vi "Robot Global Data.vi"() -> ()   [LabVIEW 2016]
doc: "This global VI can contain as many global variables as you need. Place a control on the panel, give it a good name. To read or write to it from a VI, drag the icon to the diagram of that VI. You can also drag from the project. Click on the node to change which global you access. You shouldn't have multiple locations writing to a global or it will cause a race-condition."
uses:
  <vilib>/Rock Robotics/WPI/Camera/WPI_CameraImageSize.ctl
  <vilib>/Rock Robotics/WPI/DriverStation/WPI_DriverStationRobotMode2.ctl
  Common Code/Dashboard Control Data.ctl
  Common Code/Drivetrain Settings.ctl
  Common Code/PID Gains.ctl
  Common Code/Input Modifier.ctl
  Common Code/Intake Presets.ctl
  Common Code/Shooter Presets.ctl
  Common Code/Vision Target Packet.ctl
  Common Code/Drivetrain Encoder Values.ctl
  Common Code/Encoder Values.ctl
  Common Code/Auto Agitator Settings.ctl
  Common Code/Climber Settings.ctl
  Common Code/LED Global Data.ctl
  Common Code/Drivetrain Command Cluster.ctl
  Common Code/Drivetrain Mode.ctl
  Common Code/Intake Control Cluster.ctl
  Common Code/Intake Modes.ctl
  Common Code/Intake Auto States.ctl
  Common Code/Intake Trip States.ctl
  Common Code/Keyboard Packet.ctl
  Common Code/Manual Command Cluster.ctl
  Common Code/Shooter Control Cluster'.ctl
  Common Code/Shooter Modes.ctl
  Common Code/Shooter Commands.ctl
  Common Code/Manual Shoot Cluster.ctl
  Common Code/Shot Type.ctl
  Common Code/Auton File Lists.ctl
  Common Code/Auton Command Cluster.ctl
  Common Code/Climb Command Cluster.ctl
  Common Code/Drivetrain Status Cluster.ctl
  Common Code/Intake Status Cluster.ctl
  Common Code/Climb Status Cluster.ctl
  Common Code/Shooter Status Cluster.ctl
  Common Code/Dashboard Display Data.ctl
  Common Code/Shooter Motor Operational Status .ctl
  <vilib>/Analysis/Matrix/Datatypes/RealMatrix.ctl
  Common Code/PDP Status Cluster.ctl
  Common Code/Robot Status Cluster.ctl
  <vilib>/Rock Robotics/WPI/DriverStation/WPI_DriverStationAllianceInfo.ctl
  <vilib>/Rock Robotics/WPI/DriverStation/WPI_DriverStationPositionInfo.ctl
  Common Code/Goal Vision Packet.ctl
  Common Code/Auto Agitator Control Cluster.ctl
  <vilib>/Analysis/Matrix/NI_Matrix.lvlib
panel:
  in  "Robot Status Cluster":T1
  out "PDP Status Cluster":T5
  out "Climber Tripped?":bool
  in  "Vision Presets":T6
  out "Auto Agitator Control Cluster":T7
  in  "Motor Operational Status":T8
  out "Auton Loop Timer":dbl
  out "Goal Vision Packet":T9
  in  "Dashboard Status Data":T10={"Climb Status Cluster"={"Climb Speed"=0.0}, "Drivetrain Status Cluster"={"Drivetrain Mode"=enum."Manual", "Y (Throttle)"=0.0, "X (Steer)"=0.0, "Z (Strafe)"=0.0, "Heading Target"=0.0, "Center Piston Down?"=FALSE, "Traction?"=FALSE, "Gyro Steer Finished?"=FALSE, "Distance Drive Finished?"=FALSE, "Gyro"=0.0, "Distance Target"=0.0, "Y Max Output"=0.0, "Y Min Output"=0.0, "X Max Output"=0.0, "X Min Output"=0.0, "Z Max Output"=0.0, "Z Min Output"=0.0, "Translation Target"=0.0, "Translation Drive Finished?"=FALSE, "PID Auto Drive Finished?"=FALSE, "Brake?"=FALSE, "Vision Aligned?"=FALSE, "Creep Mode Engaged?"=FALSE}, "Intake Status Cluster"={"Roller Power"=0.0, "Intake Mode"=enum."Manual", "Intake Auto State"=enum."Idle", "Backward Tripped?"=FALSE, "Forward Tripped?"=FALSE, "Intake Current Trip State"=enum."Normal", "Gear Slot Open"=FALSE, "Wings Open"=FALSE, "Traction for Gear?"=FALSE, "Current Over Max Current?"=FALSE, "Tripped?"=FALSE, "Current"=0.0, "Intake Down?"=FALSE, "Gear Loaded"=FALSE}, "Shooter Status Cluster"={"Current RPM"=0.0, "Trigger Power"=0.0, "Shooter Mode"=enum."Auto", "Shot Type"=enum."Dist Shot", "Shooter State"=enum."Idle ", "Target RPM"=0.0, "Hood Down?"=FALSE, "RPM Reached?"=FALSE, "User Inputed RPM"=0.0}, "Drivetrain Encoder Values"={"Left Encoder"={"Distance"=0.0, "Speed"=0.0, "Tick"=0.0}, "Center Encoder"={"Distance"=0.0, "Speed"=0.0, "Tick"=0.0}, "Right Encoder"={"Distance"=0.0, "Speed"=0.0, "Tick"=0.0}}, "Auton Command Cluster"={"commandID"=0.0, "maxTime"=0.0, "distanceTarget"=0.0, "headingTarget"=0.0, "translationTarget"=0.0, "ySpeed"=0.0, "xSpeed"=0.0, "zSpeed"=0.0, "async"=0.0, "shotType"=0.0, "shootCommand"=0.0, "rollerPower"=0.0, "fillHopper?"=0.0, "zeroGyro"=0.0, "openGear"=0.0, "traction?"=0.0}, "Auton File Lists"={"Current Queue"="", "General Scripts"="", "Movements"=""}, "Pressure"=0.0, "Pressure Voltage"=0.0, "Motor Operational Status"={"Sensor Velocity "=0.0, "Encoder Position"=0.0, "Encoder Velocity "=0.0, "Encoder Index Count"=0.0, "Analog In"=0.0, "Analog In Velocity"=0.0, "Battery Voltage"=0.0, "Current"=0.0, "Sensor Position"=0.0, "Vel Div 4"=FALSE, "Encoder A Pin State"=FALSE, "Encoder B Pin State"=FALSE, "Encoder Index Pin State"=FALSE, "Pulse Width Velocity "=0.0}, "Vision Presets"=[], "Climber Current Tripped?"=FALSE, "Gear?"=FALSE, "PDP Status Cluster"={"Drivetrain Left CIM 1"=0.0, "Drivetrain Left CIM 2"=0.0, "Drivetrain Left Mini CIM"=0.0, "Drivetrain Right CIM 1"=0.0, "Drivetrain Right CIM 2"=0.0, "Drivetrain Right Mini CIM"=0.0, "Drivetrain Center CIM 1"=0.0, "Drivetrain Center CIM 2"=0.0, "Shooter Motor 1"=0.0, "Shooter Motor 2"=0.0, "Climber Motor 1"=0.0, "Climber Motor 2"=0.0, "Intake Motor"=0.0, "Trigger Motor"=0.0, "Fans/Compressor"=0.0}, "Robot Status Cluster"={"RobotMode"=enum."Autonomous Disabled", "Alliance"=enum."Red", "Position"=enum."1", "Match Time"=0.0, "FMS?"=FALSE}} {"Shooter Status Cluster"."Current RPM" scale=0.0..5000.0; "Drivetrain Status Cluster"."Gyro" scale=180.0..-180.0}
  in  "Auton Command Cluster":T23
  in  "Shooter Status Cluster":T17={"Current RPM"=0.0, "Trigger Power"=0.0, "Shooter Mode"=enum."Auto", "Shot Type"=enum."Dist Shot", "Shooter State"=enum."Idle ", "Target RPM"=0.0, "Hood Down?"=FALSE, "RPM Reached?"=FALSE, "User Inputed RPM"=0.0} {"Current RPM" scale=0.0..5000.0}
  in  "Climb Status Cluster":T11
  in  "Intake Status Cluster":T13={"Roller Power"=0.0, "Intake Mode"=enum."Manual", "Intake Auto State"=enum."Idle", "Backward Tripped?"=FALSE, "Forward Tripped?"=FALSE, "Intake Current Trip State"=enum."Normal", "Gear Slot Open"=FALSE, "Wings Open"=FALSE, "Traction for Gear?"=FALSE, "Current Over Max Current?"=FALSE, "Tripped?"=FALSE, "Current"=0.0, "Intake Down?"=FALSE, "Gear Loaded"=FALSE}
  in  "Drivetrain Status Cluster":T12 {"Gyro" scale=180.0..-180.0}
  in  "Climb Command Cluster":T25
  in  "Drivetrain Encoder Values":T21
  in  "Auton Line Number":dbl
  in  "Auton Command Array":T23[](array[typedef])
  in  "Auton File Lists":T24
  in  "Auton File Index":i32
  in  "Queue File Names":string[](array[string])
  in  "Auton File Build Loops":i32
  in  "Auton Field Index":i32
  in  "Auton File Queue":path[](array[path])
  in  "Shooter Control Cluster":T26={"Shooter Modes"=enum."Auto", "Shooter Commands"=enum."Idle ", "Manual Control Cluster"={"Shooter Power"=0.0, "Hood Down?"=FALSE, "Trigger Power"=0.0}, "Shot Type"=enum."Dist Shot", "Agitator Power"=0.0, "Universal Modifier"=FALSE}
  in  "Manual Command Cluster":T28
  in  "Keyboard Cluster":T29
  in  "Intake Control Cluster":T30={"Intake Mode"=enum."Manual", "Intake Auto Command"=enum."Idle", "Intake Current Trip State"=enum."Normal", "Gear slot open?"=FALSE, "Engage traction for gear load?"=FALSE, "Wings open?"=FALSE, "Manual Intake Power"=0.0}
  in  "Drivetrain Command Cluster":T31
  in  "Dashboard Packet":T33={"Drivetrain Settings"={"Gyro Tolerance"=0.0, "Gyro Steer PID Gains"={"proportional gain (Kc)"=0.03, "integral time (Ti, min)"=0.01, "derivative time (Td, min)"=0.0}, "Y Power Multiplier"=6.0, "Turn Power Multiplier"=5.0, "Gyro Output"=0.85, "Creep Rate"=0.4, "Distance Drive PID Gains"={"proportional gain (Kc)"=1.0, "integral time (Ti, min)"=0.01, "derivative time (Td, min)"=0.0}, "Distance Tolerance"=1.4999999999999998, "Distance Output"=0.85, "Strafe Threshold"=0.4, "Strafe Correct"=FALSE, "Strafe Tolerance"=0.0, "Translate Drive PID Gains"={"proportional gain (Kc)"=1.0, "integral time (Ti, min)"=0.01, "derivative time (Td, min)"=0.0}, "Strafe Output"=0.0, "SC Right"=0.85, "SC Left"=0.85, "Use Gyro"=FALSE, "Constant Power"=FALSE, "Strafe Power"=0.0, "Input Modifier"=enum."None", "SCR Delay"=0.85, "SCL Delay"=0.85}, "Intake Presets "={"Intake Speed "=0.0, "Outake Speed"=0.0, "Current Trip Delay"=0.0, "Max Current"=0.0, "Gear Outtake Motor Delay"=0.0, "Gear Intake Motor Delay"=0.0, "Gear Intake?"=FALSE, "Gear Intake Pull Up Speed"=0.0}, "Shooter Presets"={"Key Shot"={"RPM "=0.0, "Hood?"=FALSE}, "Distance Shot"={"RPM"=0.0, "Hood?"=FALSE}, "RPM Tolerance"=0.0, "Unstuck Delay Time "=0.0, "Initial RPM Increase"=0.0, "Warmup Delay"=0.0, "Faster Time"=0.0, "Shooter PID Gains"={"P"=0.0, "I"=0.0, "D"=0.0, "FF"=0.0, "Ramp Rate"=0.0, "I Zone"=0.0}, "Unstuck Trigger Power"=0.0, "Trigger Power"=0.0, "Unstuck RPM"=0.0, "Agitator Active Power"=0.0, "Agitator Idle Power"=0.0, "RPM Tuning Range"=0.0, "RPM M Tuning Range"=0.0}, "Vision Target Packet"={"Robot Center"=0.0, "Center X"=0.0, "Center Y"=0.0, "Angle"=0.0, "Distance"=0.0, "Found Target?"=FALSE}, "Auton Presets"={"Start Position"=0.0}, "Drivetrain Encoder Values"={"Left Encoder"={"Distance"=0.0, "Speed"=0.0, "Tick"=0.0}, "Center Encoder"={"Distance"=0.0, "Speed"=0.0, "Tick"=0.0}, "Right Encoder"={"Distance"=0.0, "Speed"=0.0, "Tick"=0.0}}, "Drivetrain Encoder Settings"={"Left Tick Constant"=0.0, "Right Tick Contant"=0.0, "Reset Encoders"=FALSE, "Center Tick Constant"=0.0}, "Zero Gyro"=FALSE, "Vision Timeout"=0.0, "Pressure M"=0.0, "Pressure B"=0.0, "Auto Agitator"={"Enable Auto Agitation"=FALSE, "Continuous Stir"=FALSE, "Continuous Intake"=FALSE, "Alternate In/Outtake"=FALSE, "Wing Delay"=0.0, "Stir Delay"=0.0, "Intake Delay"=0.0, "Wing On Time"=0.0, "Wing Off Time"=0.0, "Stir On Time"=0.0, "Stir Off Time"=0.0, "Intake On Time"=0.0, "Intake Off Time"=0.0, "Stir Power"=0.0, "Intake Power"=0.0, "Outtake Power"=0.0, "Intake Run Time"=0.0, "Outtake Run Time"=0.0, "Wing$"=FALSE, "Intake"=FALSE, "Stirrer"=FALSE}, "Climber Settings"={"Climber Power"=0.0, "Max Current"=0.0, "Avoid Current Trip?"=FALSE}, "LEDs"={"Back"={"Default"="", "Traction"="", "Gear Ready"="", "Break On"="", "Gear Loaded"=""}, "Front"={"Default"="", "Traction"="", "Gear Ready"="", "Break On"="", "Gear Loaded"=""}}} {"Shooter Presets"."Shooter PID Gains"."D" format="%.3f"; "Shooter Presets"."Shooter PID Gains"."I" format="%.3f"; "Shooter Presets"."Shooter PID Gains"."P" format="%.3f"; "Drivetrain Settings"."Translate Drive PID Gains"."derivative time (Td, min)" format="%.3f"; "Drivetrain Settings"."Translate Drive PID Gains"."integral time (Ti, min)" format="%.3f"; "Drivetrain Settings"."Translate Drive PID Gains"."proportional gain (Kc)" format="%.3f"; "Drivetrain Settings"."Distance Drive PID Gains"."derivative time (Td, min)" format="%.3f"; "Drivetrain Settings"."Distance Drive PID Gains"."integral time (Ti, min)" format="%.3f"; "Drivetrain Settings"."Distance Drive PID Gains"."proportional gain (Kc)" format="%.3f"; "Drivetrain Settings"."Turn Power Multiplier" scale=0.0..6.0; "Drivetrain Settings"."Y Power Multiplier" scale=0.0..6.0; "Drivetrain Settings"."Gyro Steer PID Gains"."derivative time (Td, min)" format="%.3f"; "Drivetrain Settings"."Gyro Steer PID Gains"."integral time (Ti, min)" format="%.3f"; "Drivetrain Settings"."Gyro Steer PID Gains"."proportional gain (Kc)" format="%.3f"}
  out "Driver Station IP":dbl
  in  "Robot Mode":T2
  in  "image size":T43=enum."320x240"
  in  "Enable Vision":bool
  # "Auton"
  # "Dashboard"
  # "Drivetrain"
  # "Shooter"
  # "Intake"
  # "Climber"
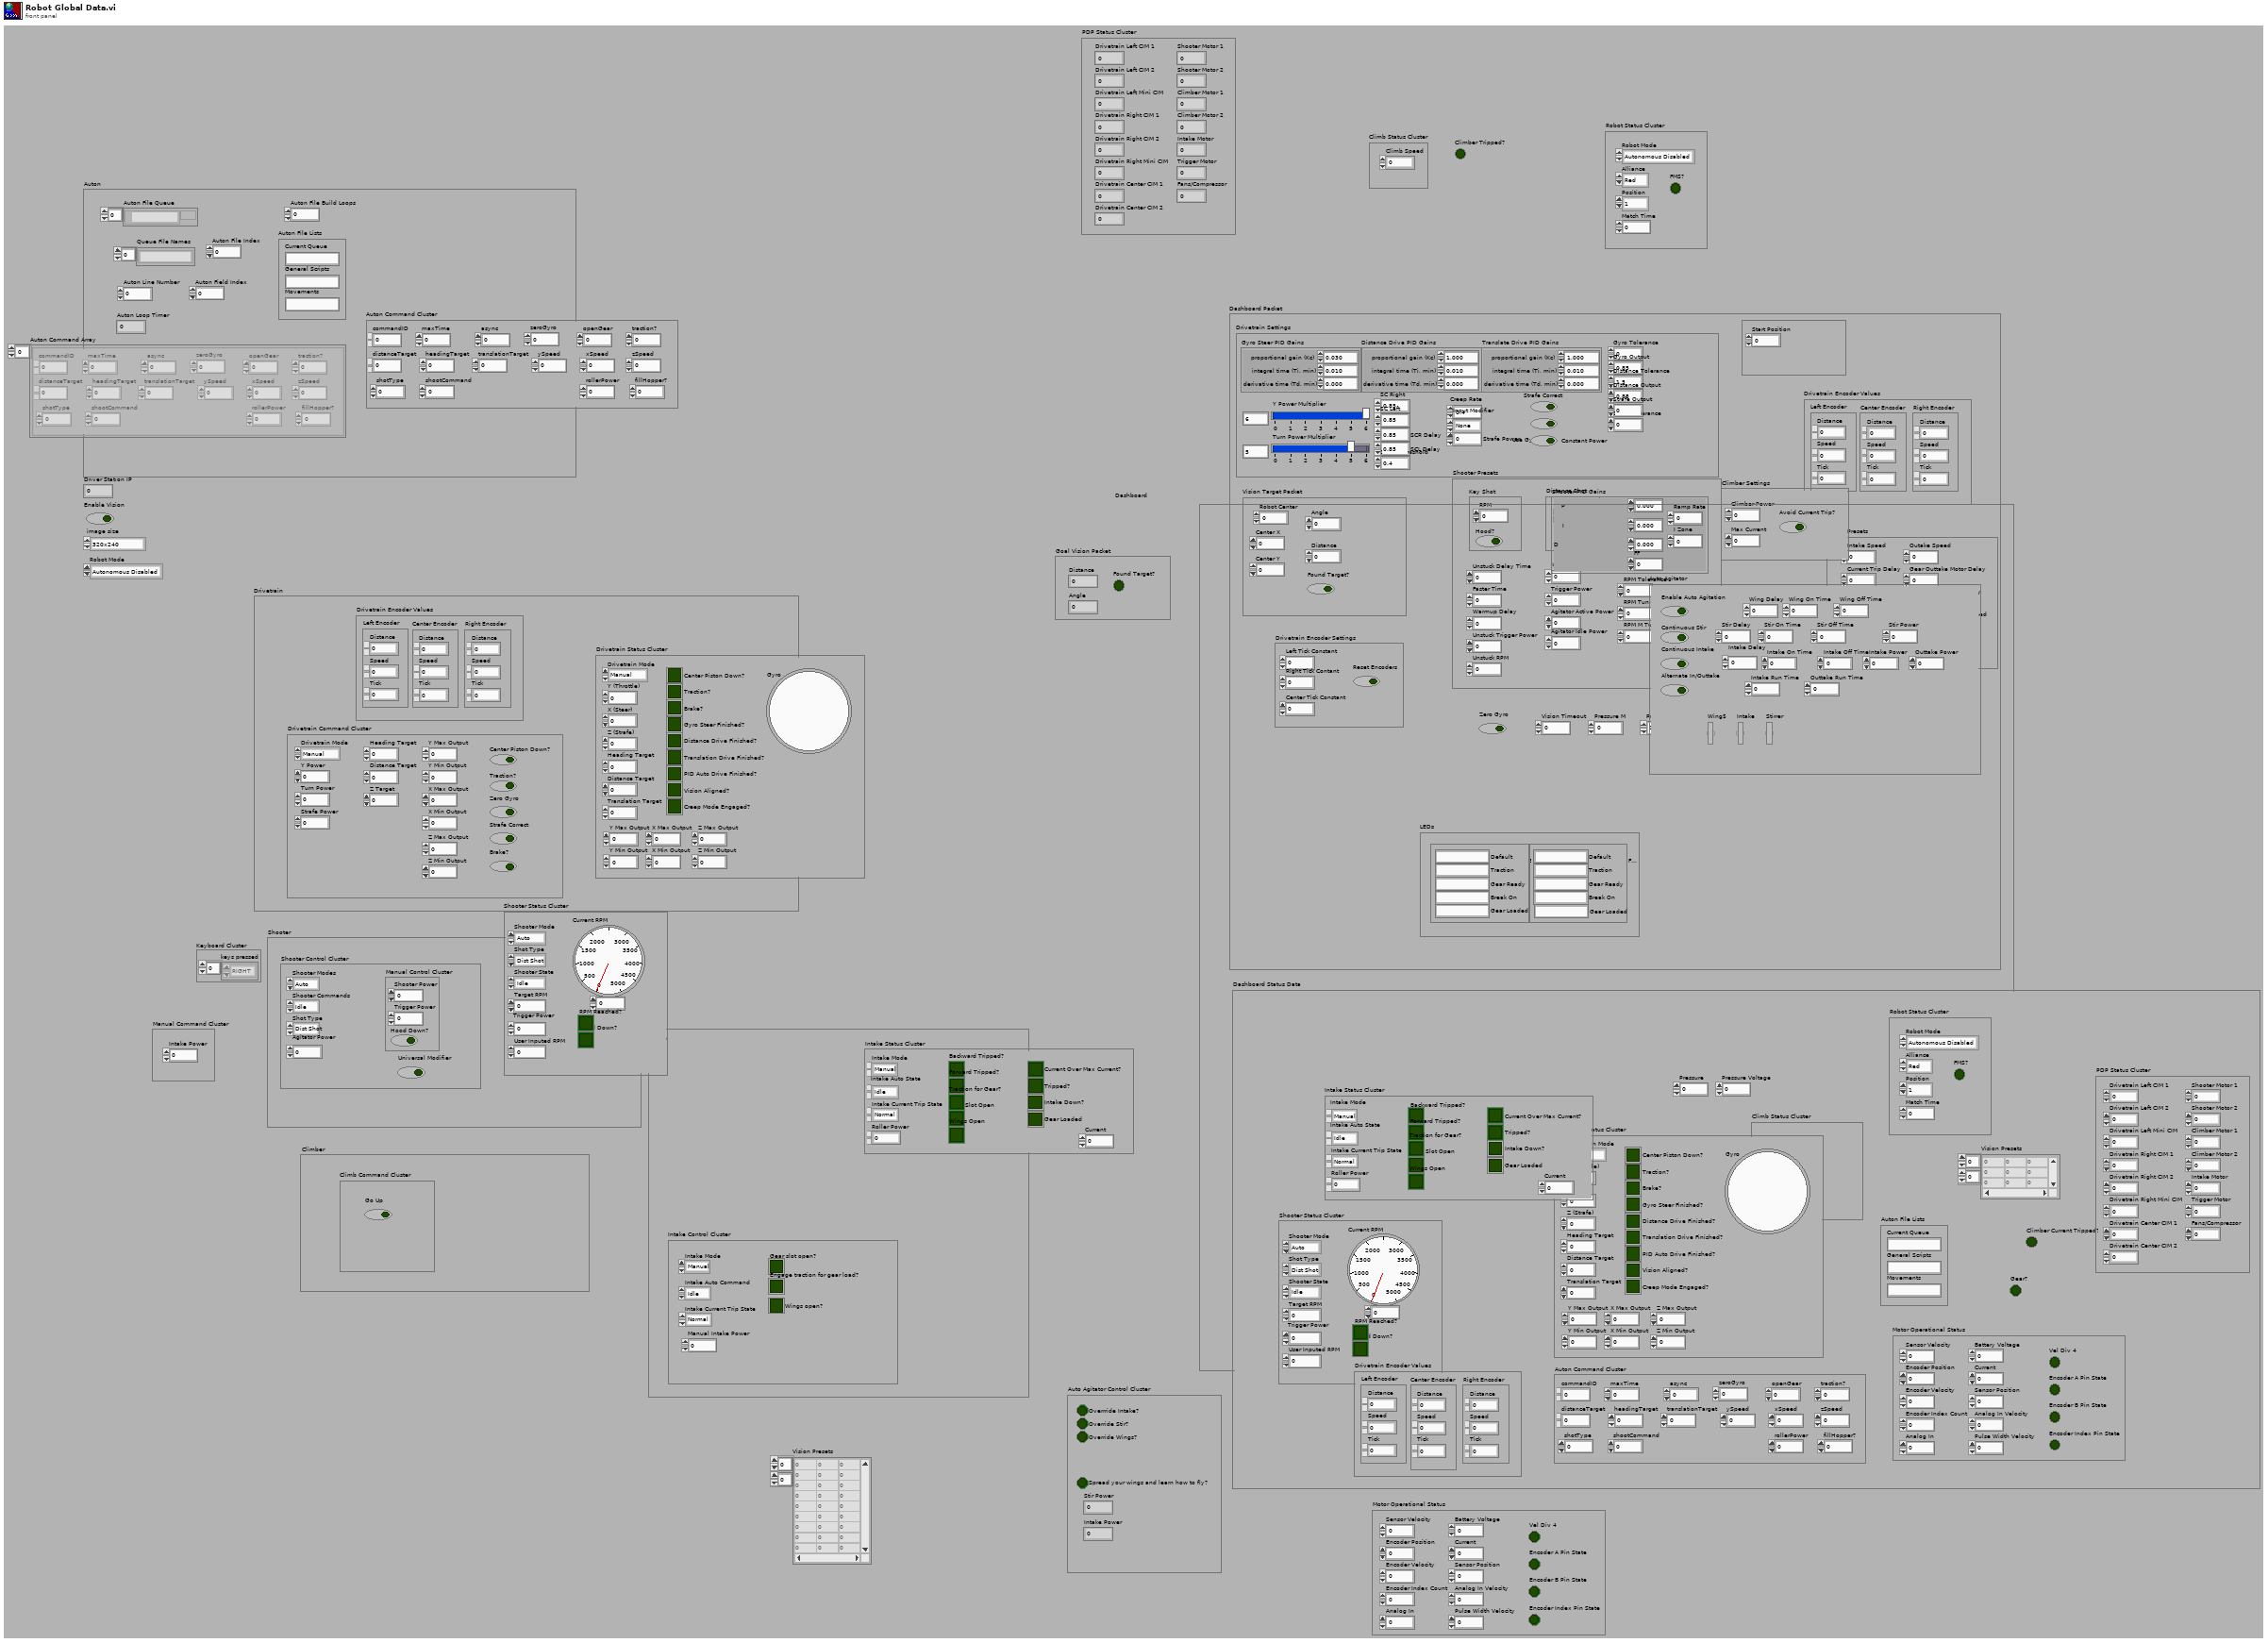
[diagram p1: front panel]
types:
  T1 = typedef "Robot Status Cluster.ctl" = cluster{"RobotMode":T2, "Alliance":T3, "Position":T4, "Match Time":dbl, "FMS?":bool}
  T2 = typedef "WPI_DriverStationRobotMode2.ctl" = enum16{"Autonomous Disabled", "Autonomous Enabled", "Teleop Disabled", "Teleop Enabled", "Disconnected", "Finish", "Test Disabled", "Test Enabled", "Emergency Stopped"}
  T3 = typedef "WPI_DriverStationAllianceInfo.ctl" = enum16{"Red", "Blue", "Invalid"}
  T4 = typedef "WPI_DriverStationPositionInfo.ctl" = enum16{"1", "2", "3"}
  T5 = typedef "PDP Status Cluster.ctl" = cluster{"Drivetrain Left CIM 1":dbl, "Drivetrain Left CIM 2":dbl, "Drivetrain Left Mini CIM":dbl, "Drivetrain Right CIM 1":dbl, "Drivetrain Right CIM 2":dbl, "Drivetrain Right Mini CIM":dbl, "Drivetrain Center CIM 1":dbl, "Drivetrain Center CIM 2":dbl, "Shooter Motor 1":dbl, "Shooter Motor 2":dbl, "Climber Motor 1":dbl, "Climber Motor 2":dbl, "Intake Motor":dbl, "Trigger Motor":dbl, "Fans/Compressor":dbl}
  T6 = typedef "NI_Matrix.lvlib/RealMatrix.ctl" = dbl[][]
  T7 = typedef "Auto Agitator Control Cluster.ctl" = cluster{"Overrride Intake?":bool, "Spread your wings and learn how to fly?":bool, "Stir Power":dbl, "Intake Power":dbl, "Override Stir?":bool, "Override Wings?":bool}
  T8 = typedef "Shooter Motor Operational Status .ctl" = cluster{"Sensor Velocity ":dbl, "Encoder Position":dbl, "Encoder Velocity ":dbl, "Encoder Index Count":dbl, "Analog In":dbl, "Analog In Velocity":dbl, "Battery Voltage":dbl, "Current":dbl, "Sensor Position":dbl, "Vel Div 4":bool, "Encoder A Pin State":bool, "Encoder B Pin State":bool, "Encoder Index Pin State":bool, "Pulse Width Velocity ":dbl}
  T9 = typedef "Goal Vision Packet.ctl" = cluster{"Distance":dbl, "Angle":dbl, "Found Target?":bool}
  T10 = typedef "Dashboard Display Data.ctl" = cluster{"Climb Status Cluster":T11, "Drivetrain Status Cluster":T12, "Intake Status Cluster":T13, "Shooter Status Cluster":T17, "Drivetrain Encoder Values":T21, "Auton Command Cluster":T23, "Auton File Lists":T24, "Pressure":dbl, "Pressure Voltage":dbl, "Motor Operational Status":T8, "Vision Presets":T6, "Climber Current Tripped?":bool, "Gear?":bool, "PDP Status Cluster":T5, "Robot Status Cluster":T1}
  T11 = typedef "Climb Status Cluster.ctl" = cluster{"Climb Speed":dbl}
  T12 = typedef "Drivetrain Status Cluster.ctl" = cluster{"Drivetrain Mode":enum16{"Manual", "Gyro Steer"}, "Y (Throttle)":dbl, "X (Steer)":dbl, "Z (Strafe)":dbl, "Heading Target":dbl, "Center Piston Down?":bool, "Traction?":bool, "Gyro Steer Finished?":bool, "Distance Drive Finished?":bool, "Gyro":dbl, "Distance Target":dbl, "Y Max Output":dbl, "Y Min Output":dbl, "X Max Output":dbl, "X Min Output":dbl, "Z Max Output":dbl, "Z Min Output":dbl, "Translation Target":dbl, "Translation Drive Finished?":bool, "PID Auto Drive Finished?":bool, "Brake?":bool, "Vision Aligned?":bool, "Creep Mode Engaged?":bool}
  T13 = typedef "Intake Status Cluster.ctl" = cluster{"Roller Power":dbl, "Intake Mode":T14, "Intake Auto State":T15, "Backward Tripped?":bool, "Forward Tripped?":bool, "Intake Current Trip State":T16, "Gear Slot Open":bool, "Wings Open":bool, "Traction for Gear?":bool, "Current Over Max Current?":bool, "Tripped?":bool, "Current":dbl, "Intake Down?":bool, "Gear Loaded":bool}
  T14 = typedef "Intake Modes.ctl" = enum16{"Manual", "Auto"}
  T15 = typedef "Intake Auto States.ctl" = enum16{"Outtake", "Idle", "Intake", "Intake Pull Up"}
  T16 = typedef "Intake Trip States.ctl" = enum16{"Normal", "Backward Tripped", "Forward Tripped"}
  T17 = typedef "Shooter Status Cluster.ctl" = cluster{"Current RPM":dbl, "Trigger Power":dbl, "Shooter Mode":T18, "Shot Type":T19, "Shooter State":T20, "Target RPM":dbl, "Hood Down?":bool, "RPM Reached?":bool, "User Inputed RPM":dbl}
  T18 = typedef "Shooter Modes.ctl" = enum16{"Auto", "Manual"}
  T19 = typedef "Shot Type.ctl" = enum16{"Vision Shot", "Dist Shot", "Key Shot"}
  T20 = typedef "Shooter Commands.ctl" = enum16{"Idle ", "Warmup ", "Shoot"}
  T21 = typedef "Drivetrain Encoder Values.ctl" = cluster{"Left Encoder":T22, "Center Encoder":T22, "Right Encoder":T22}
  T22 = typedef "Encoder Values.ctl" = cluster{"Distance":dbl, "Speed":dbl, "Tick":dbl}
  T23 = typedef "Auton Command Cluster.ctl" = cluster{"commandID":dbl, "maxTime":dbl, "distanceTarget":dbl, "headingTarget":dbl, "translationTarget":dbl, "ySpeed":dbl, "xSpeed":dbl, "zSpeed":dbl, "async":dbl, "shotType":dbl, "shootCommand":dbl, "rollerPower":dbl, "fillHopper?":dbl, "zeroGyro":dbl, "openGear":dbl, "traction?":dbl}
  T24 = typedef "Auton File Lists.ctl" = cluster{"Current Queue":string, "General Scripts":string, "Movements":string}
  T25 = typedef "Climb Command Cluster.ctl" = cluster{"Go Up":bool}
  T26 = typedef "Shooter Control Cluster'.ctl" = cluster{"Shooter Modes":T18, "Shooter Commands":T20, "Manual Control Cluster":T27, "Shot Type":T19, "Agitator Power":dbl, "Universal Modifier":bool}
  T27 = typedef "Manual Shoot Cluster.ctl" = cluster{"Shooter Power":dbl, "Hood Down?":bool, "Trigger Power":dbl}
  T28 = typedef "Manual Command Cluster.ctl" = cluster{"Intake Power":dbl}
  T29 = typedef "Keyboard Packet.ctl" = cluster{"keys pressed":enum16{"0", "1", "2", "3", "4", "5", "6", "7", "8", "9", "A", "B", "C", "D", "E", "F", "G", "H", "I", "J", "K", "L", "M", "N", "O", "P", "Q", "R", "S", "T", "U", "V", "W", "X", "Y", "Z", "F1", "F2", "F3", "F4", "F5", "F6", "F7", "F8", "F9", "F10", "F11", "F12", "F13", "F14", "F15", "ADD", "BACK", "BACKSLASH", "CAPITAL", "COMMA", "DECIMAL", "DELETE", "DIVIDE", "DOWN", "END", "EQUALS", "ESCAPE", "GRAVE (`)", "HOME", "INSERT", "LBRACKET", "LCONTROL", "LEFT", "L ALT", "LSHIFT", "LWIN", "MINUS", "MULTIPLY", "NEXT", "NUMLOCK", "NUMPAD_0", "NUMPAD_1", "NUMPAD_2", "NUMPAD_3", "NUMPAD_4", "NUMPAD_5", "NUMPAD_6", "NUMPAD_7", "NUMPAD_8", "NUMPAD_9", "PAUSE", "PERIOD", "PRIOR (PG UP)", "RBRACKET", "RCONTROL", "RETURN", "RIGHT", "R ALT", "RSHIFT", "RWIN", "SCROLL", "SEMICOLON", "SLASH", "SPACE", "SUBTRACT", "TAB", "UP", "ENTER (num pad)", "' (quote)"}[]}
  T30 = typedef "Intake Control Cluster.ctl" = cluster{"Intake Mode":T14, "Intake Auto Command":T15, "Intake Current Trip State":T16, "Gear slot open?":bool, "Engage traction for gear load?":bool, "Wings open?":bool, "Manual Intake Power":dbl}
  T31 = typedef "Drivetrain Command Cluster.ctl" = cluster{"Drivetrain Mode":T32, "Heading Target":dbl, "Turn Power":dbl, "Y Power":dbl, "Center Piston Down?":bool, "Traction?":bool, "Strafe Power":dbl, "Zero Gyro":bool, "Distance Target":dbl, "Strafe Correct":bool, "Y Max Output":dbl, "Y Min Output":dbl, "X Max Output":dbl, "X Min Output":dbl, "Z Max Output":dbl, "Z Min Output":dbl, "Z Target":dbl, "Brake?":bool}
  T32 = typedef "Drivetrain Mode.ctl" = enum16{"Manual", "Gyro Steer", "Distance Drive", "Translate Drive", "Goal Vision Align", "PID Drive"}
  T33 = typedef "Dashboard Control Data.ctl" = cluster{"Drivetrain Settings":T34, "Intake Presets ":T37, "Shooter Presets":T38, "Vision Target Packet":T39, "Auton Presets":cluster{"Start Position":dbl}, "Drivetrain Encoder Values":T21, "Drivetrain Encoder Settings":cluster{"Left Tick Constant":dbl, "Right Tick Contant":dbl, "Reset Encoders":bool, "Center Tick Constant":dbl}, "Zero Gyro":bool, "Vision Timeout":dbl, "Pressure M":dbl, "Pressure B":dbl, "Auto Agitator":T40, "Climber Settings":T41, "LEDs":T42}
  T34 = typedef "Drivetrain Settings.ctl" = cluster{"Gyro Tolerance":dbl, "Gyro Steer PID Gains":T35, "Y Power Multiplier":dbl, "Turn Power Multiplier":dbl, "Gyro Output":dbl, "Creep Rate":dbl, "Distance Drive PID Gains":T35, "Distance Tolerance":dbl, "Distance Output":dbl, "Strafe Threshold":dbl, "Strafe Correct":bool, "Strafe Tolerance":dbl, "Translate Drive PID Gains":T35, "Strafe Output":dbl, "SC Right":dbl, "SC Left":dbl, "Use Gyro":bool, "Constant Power":bool, "Strafe Power":dbl, "Input Modifier":T36, "SCR Delay":dbl, "SCL Delay":dbl}
  T35 = typedef "PID Gains.ctl" = cluster{"proportional gain (Kc)":dbl, "integral time (Ti, min)":dbl, "derivative time (Td, min)":dbl}
  T36 = typedef "Input Modifier.ctl" = enum16{"None", "Square", "Cube"}
  T37 = typedef "Intake Presets.ctl" = cluster{"Intake Speed ":dbl, "Outake Speed":dbl, "Current Trip Delay":dbl, "Max Current":dbl, "Gear Outtake Motor Delay":dbl, "Gear Intake Motor Delay":dbl, "Gear Intake?":bool, "Gear Intake Pull Up Speed":dbl}
  T38 = typedef "Shooter Presets.ctl" = cluster{"Key Shot":cluster{"RPM ":dbl, "Hood?":bool}, "Distance Shot":cluster{"RPM":dbl, "Hood?":bool}, "RPM Tolerance":dbl, "Unstuck Delay Time ":dbl, "Initial RPM Increase":dbl, "Warmup Delay":dbl, "Faster Time":dbl, "Shooter PID Gains":cluster{"P":dbl, "I":dbl, "D":dbl, "FF":dbl, "Ramp Rate":dbl, "I Zone":dbl}, "Unstuck Trigger Power":dbl, "Trigger Power":dbl, "Unstuck RPM":dbl, "Agitator Active Power":dbl, "Agitator Idle Power":dbl, "RPM Tuning Range":dbl, "RPM M Tuning Range":dbl}
  T39 = typedef "Vision Target Packet.ctl" = cluster{"Robot Center":dbl, "Center X":dbl, "Center Y":dbl, "Angle":dbl, "Distance":dbl, "Found Target?":bool}
  T40 = typedef "Auto Agitator Settings.ctl" = cluster{"Enable Auto Agitation":bool, "Continuous Stir":bool, "Continuous Intake":bool, "Alternate In/Outtake":bool, "Wing Delay":dbl, "Stir Delay":dbl, "Intake Delay":dbl, "Wing On Time":dbl, "Wing Off Time":dbl, "Stir On Time":dbl, "Stir Off Time":dbl, "Intake On Time":dbl, "Intake Off Time":dbl, "Stir Power":dbl, "Intake Power":dbl, "Outtake Power":dbl, "Intake Run Time":dbl, "Outtake Run Time":dbl, "Wing$":bool, "Intake":bool, "Stirrer":bool}
  T41 = typedef "Climber Settings.ctl" = cluster{"Climber Power":dbl, "Max Current":dbl, "Avoid Current Trip?":bool}
  T42 = typedef "LED Global Data.ctl" = cluster{"Back":cluster{"Default":string, "Traction":string, "Gear Ready":string, "Break On":string, "Gear Loaded":string}, "Front":cluster{"Default":string, "Traction":string, "Gear Ready":string, "Break On":string, "Gear Loaded":string}}
  T43 = typedef "WPI_CameraImageSize.ctl" = enum16{"640x480", "320x240", "160x120", "Custom"}
diagram:
